vi "Python_CMD Send Response.vi"(6 "error in (no error)":errorcluster, 7 "TCP Connection ID":T2, 8 "non-fatal error":errorcluster, 9 "Response Type":T1, 10 "Response":string, 11 "PYTHON Command String":string) -> (0 "error out":errorcluster)   [LabVIEW 2020, in "jki_python_bridge.lvlib" / "Server.lvclass"]
uses:
  Server.lvclass
  Server.lvclass/Server.ctl
  <vilib>/Utility/error.llb/DialogType.ctl
  <userlib>/_OpenG.lib/string/string.llb/openg_string.lvlib
  Python Data Tools/source/jki_python_data_tools.lvlib
  Python Data Tools/source/LabVIEW Data to Python String/LabVIEW Data to Python String (Variant).vi
  Type Definitions/PythonResponseType.ctl
  <vilib>/addons/_JKI.lib/_JKI_lib_TCP_Server.llb/TCP Server Connection Session ID Cluster.ctl
  <vilib>/addons/_JKI.lib/_JKI_lib_TCP_Server.llb/JKI TCP Server.lvclass
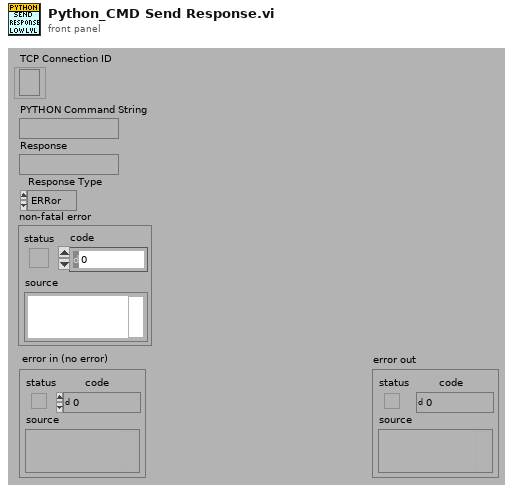
[diagram p1: front panel]
types:
  T1 = typedef "jki_python_bridge.lvlib/Server.lvclass/PythonResponseType.ctl" = enum16{"ERRor", "OK", "NEXT"}
  T2 = typedef "JKI TCP Server.lvclass/TCP Server Connection Session ID Cluster.ctl" = refnum<k5>
  T3 = typedef "DialogType.ctl" = u16
  T4 = cluster{"code out":i32, "PYTHON Command String":string, "Response":string}
  T5 = cluster{"code out":i32, "delimited string":string, "delimited string":string}
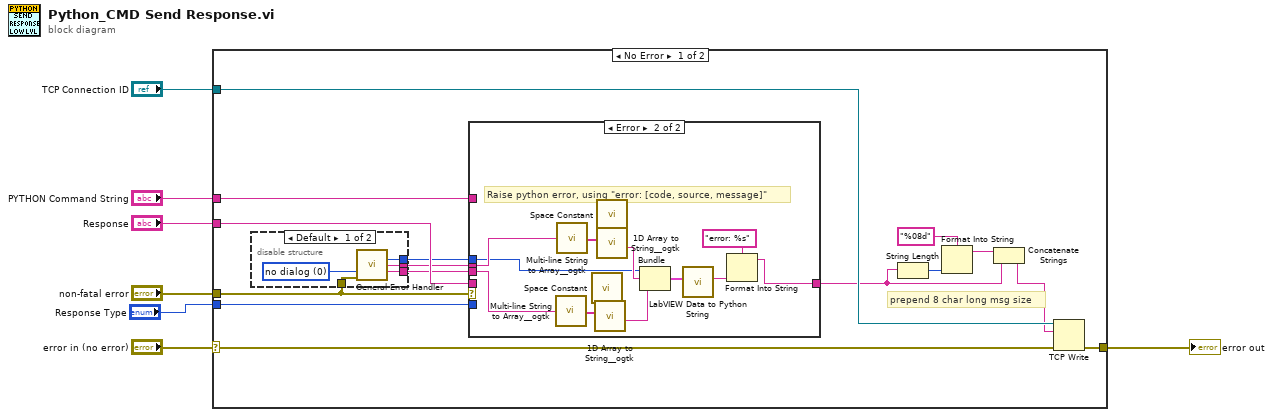
[diagram p0: block diagram]
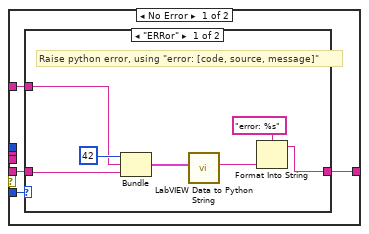
[diagram p3: hidden frame]
diagram:
  n1 = case shown="No Error" "error in (no error)" {
    selector: "error in (no error)" -> [w16 w53]
    tunnel: [w22 w53] -> w7
    tunnel: "Response Type" -> [w21 _]
    tunnel: "Response" -> [w20 _]
    tunnel: "PYTHON Command String" -> [w19 _]
    tunnel: "non-fatal error" -> [w18 _]
    tunnel: "TCP Connection ID" -> [w17 _]
    frame No Error {
      # "prepend 8 char long msg size"
      n2 = disable-structure shown="Default" {
        disable-tunnel: w18 -> [w27 _]
        disable-tunnel: [w25 _] -> w13
        disable-tunnel: [w24 _] -> w12
        disable-tunnel: [w23 _] -> w11
        frame condition #0 (active) {
          w26 = T3 0 items=["no dialog", "OK message", "continue or stop message", "OK message + warnings", "continue/stop + warnings"] ("type of dialog (OK msg:1)")
          n3 = call <vilib>:"General Error Handler.vi"("type of dialog (OK msg:1)"=w26, "error in (no error)"=w27) -> ("code out"=w23:i32, "source out"=w25:string, "message"=w24:string)  [unwired: 9 in, 2 out]
        }
        frame condition #1 {
        }
      }
      n4 = case shown="Error" w18 {
        tunnel: w20 -> [w30 _]
        tunnel: [w29 w49] -> w14
        tunnel: w13 -> [_ w42]
        tunnel: w12 -> [_ w41]
        tunnel: w11 -> [_ w40]
        tunnel: w21 -> [w31 _]
        tunnel: w19 -> [w28 _]
        frame No Error {
          n5 = case shown="\"ERRor\"" w31 {
            tunnel: w30 -> [w35 w39]
            tunnel: [w37 w39] -> w29
            tunnel: w28 -> [w34 _]
            frame "ERRor" {
              # "Raise python error, using \"error: [code, source, message]\""
              n6 = Bundle("code out"=42, "PYTHON Command String"=w34, "Response"=w35) -> (w32:T4)  [unwired: 1 in]
              n7 = call-poly "LabVIEW Data to Python String.vi"("LabVIEW Data"=w32) -> ("Python String"=w33:string)  [unwired: 9 in, 1 out]
              n8 = Format Into String(format string="error: %s", w33) -> (resulting string=w37:string)  [unwired: 2 in, 1 out]
            }
            frame Default {
            }
          }
        }
        frame Error {
          # "Raise python error, using \"error: [code, source, message]\""
          n9 = call <userlib>:"Multi-line String to Array__ogtk.vi"("string"=w41) -> ("lines"=w48:string[])
          n10 = call <userlib>:"Multi-line String to Array__ogtk.vi"("string"=w42) -> ("lines"=w44:string[])
          n11 = call <vilib>:"Space Constant.vi"() -> ("String"=w47:string)
          n12 = call <userlib>:"1D Array to String__ogtk.vi"("delimiter (Tab)"=w47, "Array of Strings"=w48) -> ("delimited string"=w46:string)  [unwired: 9 in]
          n13 = call <vilib>:"Space Constant.vi"() -> ("String"=w45:string)
          n14 = call <userlib>:"1D Array to String__ogtk.vi"("delimiter (Tab)"=w45, "Array of Strings"=w44) -> ("delimited string"=w43:string)  [unwired: 9 in]
          n15 = Bundle("code out"=w40, "delimited string"=w43, "delimited string"=w46) -> (w52:T5)  [unwired: 1 in]
          n16 = call-poly "LabVIEW Data to Python String.vi"("LabVIEW Data"=w52) -> ("Python String"=w51:string)  [unwired: 9 in, 1 out]
          n17 = Format Into String(format string="error: %s", w51) -> (resulting string=w49:string)  [unwired: 2 in, 1 out]
        }
      }
      n18 = String Length(string=w14) -> (length=w10:i32)
      n19 = Format Into String(format string="%08d", w10) -> (resulting string=w8:string)  [unwired: 2 in, 1 out]
      n20 = Concatenate Strings(w8, w14) -> (w15:string)
      n21 = TCP Write(connection ID=w17, data in=w15, error in (no error)=w16) -> (error out=w22:errorcluster)  [unwired: 1 in, 2 out]
    }
    frame Error {
    }
  }
  "error out" <- w7
